vi "Create NI 9482.vi"(8 "error in":errorcluster, 11 "channel settings":T1[](array[typedef])) -> (0 "error out":errorcluster, 3 "NI 9482 out":refnum<class "NI 9482.lvclass">)   [LabVIEW 2017, in "Scan Engine Scripting.lvlib" / "NI 9482.lvclass"]
uses:
  NI 9482.lvclass
  Mode Classes/Controls/digital channel settings.ctl
  Scan Engine Scripting.lvlib
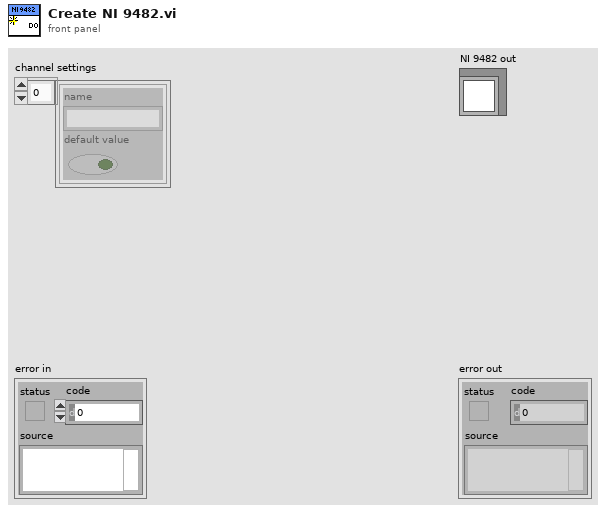
[diagram p1: front panel]
types:
  T1 = typedef "Scan Engine Scripting.lvlib/digital channel settings.ctl" = cluster{"name":string, "default value":bool}
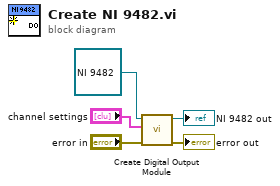
[diagram p0: block diagram]
diagram:
  n1 = call-dynamic "Create Digital Output Module.vi"("error in"="error in", "channel settings"="channel settings", "module in"=refnum<class "NI 9482.lvclass"> refnum ("NI 9482 out")) -> ("error out"=→"error out":errorcluster, "module out"=→"NI 9482 out":refnum<class "NI 9482.lvclass">)  [unwired: 7 in]
